vi "Uninitialize Interface.vi"(8 "error in (no error)":errorcluster) -> (0 "error out":errorcluster)   [LabVIEW 2019, in "Camera Engine.lvlib"]
uses:
  Camera Engine.lvlib
panel:
  # "Input"
  # "Output"
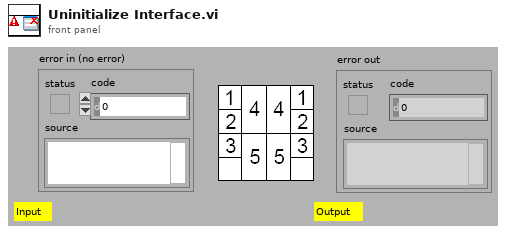
[diagram p1: front panel]
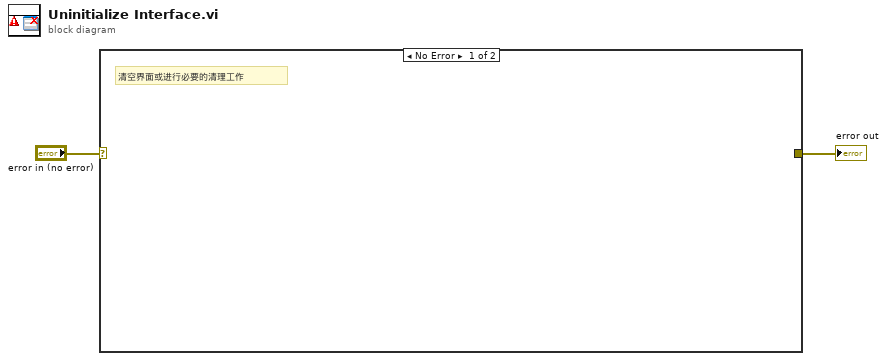
[diagram p0: block diagram]
diagram:
  n1 = case shown="No Error" "error in (no error)" {
    selector: "error in (no error)" -> [_ w3]
    tunnel: [_ w3] -> w1
    frame No Error {
      # "清空界面或进行必要的清理工作"
    }
    frame Error {
    }
  }
  "error out" <- w1
